vi "parseResetFrame.vi"(8 "error in (no error)":errorcluster, 10 "ModbusBuffer in":refnum<class "ModbusBuffer.lvclass">, 11 "ILC in":refnum<class "ILC.lvclass">) -> (0 "error out":errorcluster, 2 "ModbusBuffer out":refnum<class "ModbusBuffer.lvclass">, 3 "ILC out":refnum<class "ILC.lvclass">)   [LabVIEW 2016, in "RTILC.lvlib" / "ILC.lvclass"]
uses:
  ILC.lvclass
  Common_RT_Modbus/ModbusBuffer/ModbusBuffer.lvclass
  Common_RT_Modbus/DataTypes/ExceptionCodes.ctl
  Common_RT_Modbus/ModbusBuffer/ModbusBuffer.lvclass/ModbusBuffer.ctl
  ILC.lvclass/ILC.ctl
  Common_RT_Modbus/ModbusBuffer/readU8.vi
  Common_RT_Modbus/ModbusBuffer/readTimestampByte.vi
  Common_RT_Modbus/ModbusBuffer/readInstructionByte.vi
  Common_RT_Modbus/RTModbus.lvlib
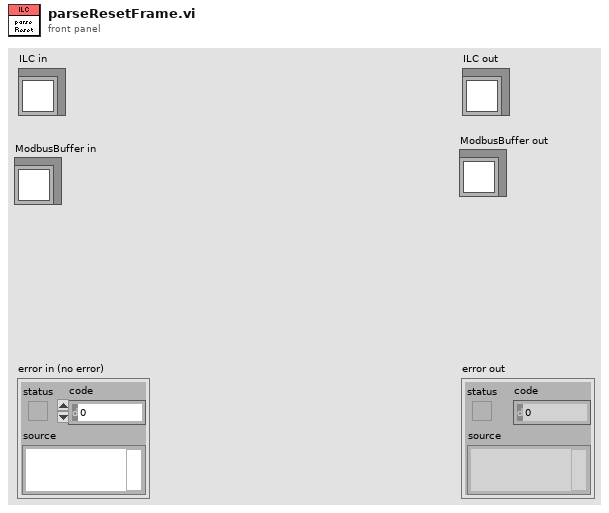
[diagram p1: front panel]
types:
  T1 = typedef "RTModbus.lvlib/ExceptionCodes.ctl" = u16
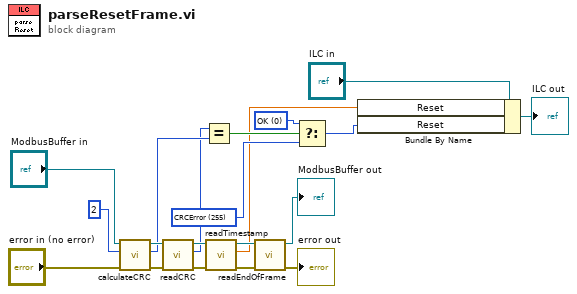
[diagram p0: block diagram]
diagram:
  w16 = T1 255 items=["OK"=0, "IllegalFunction"=1, "IllegalDataAddress"=2, "IllegalDataValue"=3, "SlaveDeviceFailure"=4, "Acknowledge"=5, "SlaveDeviceBusy"=6, "NegativeAcknowledge"=7, "MemoryParityError"=8, "GatewayPathUnavailable"=9, "GatewayTargetDeviceFailedToRespond"=10, "WaitingForResponse"=254, "CRCError"=255] ("f")
  w17 = T1 0 items=["OK"=0, "IllegalFunction"=1, "IllegalDataAddress"=2, "IllegalDataValue"=3, "SlaveDeviceFailure"=4, "Acknowledge"=5, "SlaveDeviceBusy"=6, "NegativeAcknowledge"=7, "MemoryParityError"=8, "GatewayPathUnavailable"=9, "GatewayTargetDeviceFailedToRespond"=10, "WaitingForResponse"=254, "CRCError"=255] ("Responses.ADCOffsetSensitivity")
  n1 = call "calculateCRC.vi"("error in (no error)"="error in (no error)", "Length"=u16 2, "ModbusBuffer in"="ModbusBuffer in") -> ("error out"=w10:errorcluster, "CRC"=w9:u16, "ModbusBuffer out"=w15:refnum<class "ModbusBuffer.lvclass">)  [unwired: 6 in]
  n2 = call "readCRC.vi"("error in (no error)"=w10, "ModbusBuffer in"=w15) -> ("error out"=w11:errorcluster, "Output"=w8:u16, "ModbusBuffer out"=w14:refnum<class "ModbusBuffer.lvclass">)  [unwired: 7 in]
  n3 = Equal?(x=w8, y=w9) -> (x = y?=w18:bool)
  n4 = call "readTimestamp.vi"("error in (no error)"=w11, "ModbusBuffer in"=w14) -> ("error out"=w12:errorcluster, "Output"=w5:dbl, "ModbusBuffer out"=w13:refnum<class "ModbusBuffer.lvclass">)  [unwired: 7 in]
  n5 = call "readEndOfFrame.vi"("error in (no error)"=w12, "ModbusBuffer in"=w13) -> ("error out"=→"error out":errorcluster, "ModbusBuffer out"=→"ModbusBuffer out":refnum<class "ModbusBuffer.lvclass">)  [unwired: 8 in]
  n6 = Select(t=w17, s=w18, f=w16) -> (s? t:f=w4:T1)
  n7 = Bundle By Name(cluster="ILC in", "Reset"=w5, "Reset"=w4) -> (→"ILC out":refnum<class "ILC.lvclass">)
